vi "SVFA FFT Spectrum (Complex) (1 Ch).vi"(0 "scaled signal [EU]":waveform(dbl), 2 "window":T9=8 items=["None"=0, "Hanning"=1, "Hamming"=2, "Blackman-Harris"=3, "Exact Blackman"=4, "Blackman"=5, "Flat Top"=6, "4 Term B-Harris "=7, "7 Term B-Harris"=8, "Low Sidelobe"=9, "Force"=64, "Exponential"=65, "Blackman Nuttall"=11, "Triangle"=30, "Bartlett-Hanning"=31, "Bohman"=32, "Parzen"=33, "Welch"=34, "Kaiser"=60, "Dolph-Chebyshev"=61, "Gaussian"=62], 5 "error in":errorcluster, 7 "averaging parameters":T1={"averaging mode"=enum."No averaging", "weighting mode"=enum."Exponential", "number of averages"=10, "linear mode"=enum."One shot"} {"number of averages" min=1 step=1}, 9 "restart averaging (F)":bool) -> (11 "averaging done":bool, 13 "averages completed":dbl, 14 "complex spectrum":T8={"complex spectrum response"={"f0"=0.0, "df"=1.0, "complex spectrum"=[]}, "spectrum info"={"channel name"="", "description"="", "x-axis units"=0, "spectral info"={"spectrum type"=enum."Power [Magnitude^2]", "linear/dB"=enum."linear", "window"=0, "window size"=0, "FFT size"=0}, "engineering units"=0, "custom label"="", "dB reference [EU]"=0.0, "peak units"=enum."rms", "weighting filter"=0, "spectral density?"=FALSE, "unit label"="", "spectrum skewed?"=FALSE, "complimentary spectrum units"=enum."none"}} {"spectrum info"."x-axis units" items=["Time (s)"=0, "Frequency-CB (Hz)"=1, "Frequency-CPB (Hz)"=1248, "Frequency-Arbitrary (Hz)"=2357, "Quefrency (s)"=2, "Revolutions (rev)"=3, "Order"=4, "Speed (RPM)"=11, "Speed (rad/s)"=21, "Index"=65535]; "spectrum info"."weighting filter" items=["Linear", "A-weighting", "B-weighting", "C-weighting", "ITU-R 468-4", "Dolby", "CCITT", "C-message", "Wb", "Wc", "Wd", "We", "Wf", "Wh", "Wj", "Wk", "Wm", "AES17 20 kHz lowpass", "AES17 40 kHz lowpass", "AES17 20 kHz highpass", "AES17 40 kHz highpass"]; "spectrum info"."dB reference [EU]" format="%.2f"; "spectrum info"."engineering units" items=["custom..."=0, "V"=1, "A"=21, "C"=30, "pC"=31, "s"=32, "-"=29, "Pa"=2, "N"=20, "g"=3, "m/s^2"=4, "m/s"=5, "m"=6, "mm/s"=12, "mm"=13, "micron/s"=14, "micron"=15, "in/s^2"=7, "in/s"=8, "in"=9, "mil/s"=10, "mil"=11, "rad/s^2"=16, "rad/s"=17, "rad"=18, "deg/s^2"=26, "deg/s"=27, "deg"=28, "RPM"=22, "cycle/s^2"=23, "Hz"=24, "cycle"=25, "strain"=19]; "spectrum info"."spectral info"."window" items=["None "=0, "Hanning"=1, "Hamming"=2, "Blackman-Harris"=3, "Exact Blackman"=4, "Blackman"=5, "Flat Top"=6, "4 Term B-Harris "=7, "7 Term B-Harris"=8, "Low Sidelobe"=9, "Force - Exponential"=10, "Gaussian"=62]; "complex spectrum response"."complex spectrum" format="%.2f"; "complex spectrum response"."df" format="%.2f"; "complex spectrum response"."f0" format="%.2f"}, 19 "error out":errorcluster)   [LabVIEW 2017]
doc: "Computes the Fast Fourier Transform (FFT) spectrum of <B>scaled signal [EU]</B>. This VI returns FFT results as the complex form of the FFT spectrum. Wire data to the <B>scaled signal [EU]</B> input to determine the polymorphic instance to use or manually select the instance."
uses:
  <vilib>/addons/_NISVFA/_Shared subVIs/Controls/svc_Window.ctl
  <vilib>/addons/_NISVFA/_Shared subVIs/Controls/svc_Spectrum Info.ctl
  <vilib>/addons/_NISVFA/_Shared subVIs/Controls/svc_X-Axis Units.ctl
  <vilib>/addons/_NISVFA/_Shared subVIs/Controls/svc_Spectrum Type.ctl
  <vilib>/addons/_NISVFA/_Shared subVIs/Controls/svc_Engineering Units Text Ring.ctl
  <vilib>/addons/_NISVFA/_Shared subVIs/Controls/svc_Weighting Filter Text Ring.ctl
  <vilib>/addons/_NISVFA/_Shared subVIs/Controls/svc_Complimentary Spectrum Units.ctl
  <vilib>/Analysis/2dsp.llb/Real FFT.vi
  <vilib>/Analysis/2dsp.llb/Power Spectrum (DBL).vi
  <vilib>/addons/_NISVFA/_Shared subVIs/Spectrum Averaging/svfa_No Average Array (complex).vi
  <vilib>/addons/_NISVFA/_Shared subVIs/Spectrum Averaging/svfa_Average Array (complex).vi
  <vilib>/addons/_NISVFA/_Shared subVIs/Common/sv_Get NI Property Name String.vi
  <vilib>/addons/_NISVFA/_Shared subVIs/Spectrum Averaging/svfa_No Average Array (real).vi
  <vilib>/addons/_NISVFA/_Shared subVIs/Spectrum Averaging/svfa_Average Array (real).vi
  <vilib>/addons/_NISVFA/_Shared subVIs/Spectrum Averaging/svfa_Peak Hold Array.vi
  <vilib>/addons/_NISVFA/_Shared subVIs/Windowing/svfa_Scaled Time Domain Window (Array).vi
  <vilib>/addons/_NISVFA/_Shared subVIs/Common/svc_Get SV Channel Info.vi
  <vilib>/addons/_NISVFA/_Shared subVIs/Common/svc_Spectrum Units.vi
  <vilib>/Analysis/4window.llb/Force Window.vi
  <vilib>/Analysis/4window.llb/Force Window (DBL).vi
  <vilib>/Analysis/4window.llb/Exponential Window.vi
  <vilib>/Analysis/4window.llb/Exponential Window (DBL).vi
  <vilib>/addons/_NISVFA/_Shared subVIs/Spectrum Info/sfva_Set SV Info in Spectrum Info Description.vi
  <vilib>/addons/_NISVFA/_Shared subVIs/Spectrum Info/sfva_Get SV Info from Spectrum Info Description.vi
  <vilib>/addons/_NISVFA/_Shared subVIs/Common/svc_Get Weighting Enum and Labels.vi
  <vilib>/addons/_NISVFA/_Shared subVIs/Common/svc_Unit Label Lexical Class.vi
  <vilib>/addons/_NISVFA/_Shared subVIs/Common/svc_Engineering Units to Unit Label.vi
  <vilib>/addons/_NISVFA/_Shared subVIs/Common/svc_Format Value (DBL).vi
  <vilib>/addons/_NISVFA/_Shared subVIs/Common/svc_Channel Info to Spectrum Info.vi
  <vilib>/addons/_NISVFA/_Shared subVIs/Common/svc_Unit Label to Engineering Units.vi
  <vilib>/Utility/error.llb/Error Cluster From Error Code.vi
  <vilib>/Analysis/0measdsp.llb/Scaled Time Domain Window.vi
  <vilib>/Analysis/0measdsp.llb/Scaled Time Domain Window (DBL).vi
  <vilib>/addons/_NISVFA/_Spectrum Processing/subVIs/svfa_Spectrum Info Window to windowTd Type Def.vi
  <vilib>/addons/_NISVFA/_Shared subVIs/Common/svc_Window Parameters.vi
  <vilib>/addons/_NISVFA/_Shared subVIs/Common/svc_Get Window Info.vi
  <vilib>/Analysis/NI_AALPro.lvlib
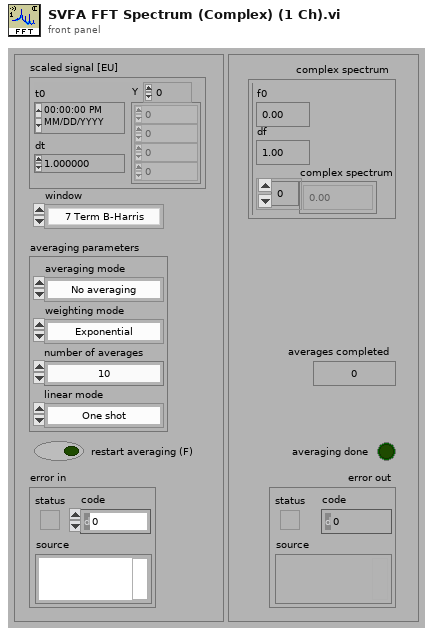
[diagram p1: front panel]
types:
  T1 = cluster{"averaging mode":enum16{"No averaging", "Vector averaging", "RMS averaging", "Peak hold"}, "weighting mode":enum16{"Linear", "Exponential"}, "number of averages":u32, "linear mode":enum16{"One shot", "Auto restart"}}
  T2 = typedef "svc_Spectrum Info.ctl" = cluster{"channel name":string, "description":string, "x-axis units":T3, "spectral info":cluster{"spectrum type":T4, "linear/dB":enum16{"linear", "dB"}, "window":u16, "window size":i32, "FFT size":i32}, "engineering units":T5, "custom label":string, "dB reference [EU]":dbl, "peak units":enum16{"rms", "peak", "peak-peak"}, "weighting filter":T6, "spectral density?":bool, "unit label":string, "spectrum skewed?":bool, "complimentary spectrum units":T7}
  T3 = typedef "svc_X-Axis Units.ctl" = u16
  T4 = typedef "svc_Spectrum Type.ctl" = enum16{"FFT Spectrum [complex]", "Amplitude [Magnitude]", "Power [Magnitude^2]", "Cross Spectrum [complex]", "Frequency Response [Complex]"}
  T5 = typedef "svc_Engineering Units Text Ring.ctl" = u16
  T6 = typedef "svc_Weighting Filter Text Ring.ctl" = u16
  T7 = typedef "svc_Complimentary Spectrum Units.ctl" = enum16{"none", "radians", "degrees", "cycles", "imaginary"}
  T8 = cluster{"complex spectrum response":cluster{"f0":dbl, "df":dbl, "complex spectrum":cdb[]}, "spectrum info":T2}
  T9 = typedef "svc_Window.ctl" = u32
  T10 = enum16{"Restart processing", "Continue processing", "Skip processing"}
  T11 = cluster{"complex FFT":cdb[], "Mag/Real FFT":dbl[], "f0":dbl, "df":dbl, "averages completed":dbl, "averaging parameters":cluster{"averaging mode":enum16{"No averaging", "Vector averaging", "RMS averaging", "Peak hold"}, "weighting mode":enum16{"Linear", "Exponential"}, "number of averages":u32, "linear mode":enum16{"One shot", "Auto restart"}}}
  T12 = enum16{"No averaging", "Vector averaging", "RMS averaging", "Peak hold"}
  T13 = cluster{"complex FFT":cdb[], "real FFT":dbl[], "f0":dbl, "df":dbl, "averages completed":dbl, "averaging parameters":cluster{"averaging mode":enum16{"No averaging", "Vector averaging", "RMS averaging", "Peak hold"}, "weighting mode":enum16{"Linear", "Exponential"}, "number of averages":u32, "linear mode":enum16{"One shot", "Auto restart"}}}
  T14 = cluster{"complex spectrum":cluster{"f0":dbl, "df":dbl, "complex spectrum":cdb[]}, "spectrum info":T2}
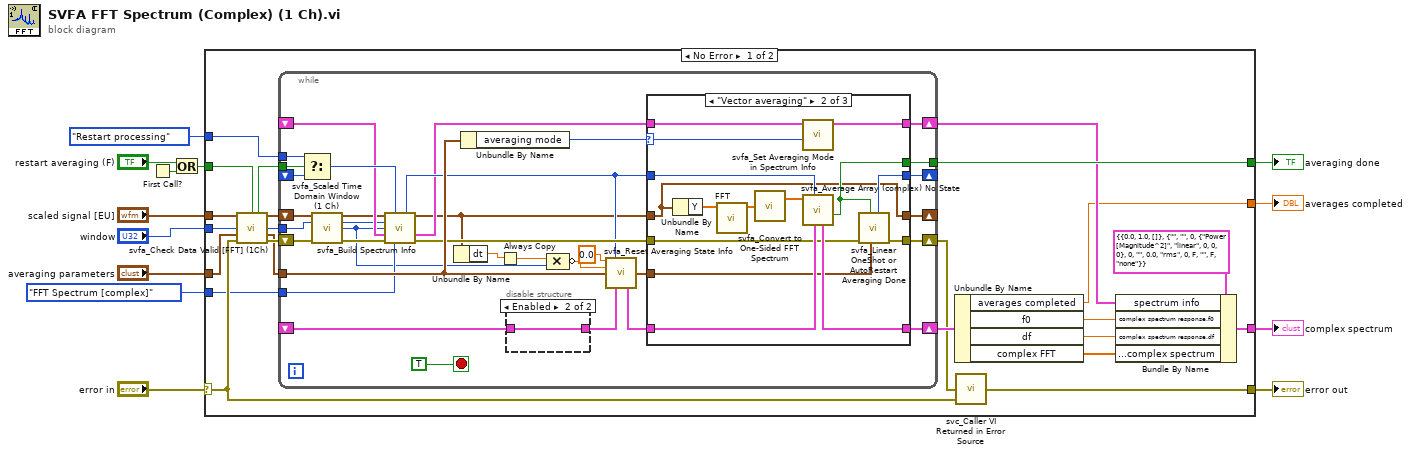
[diagram p0: block diagram]
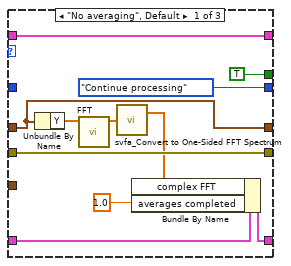
[diagram p2: hidden frame]
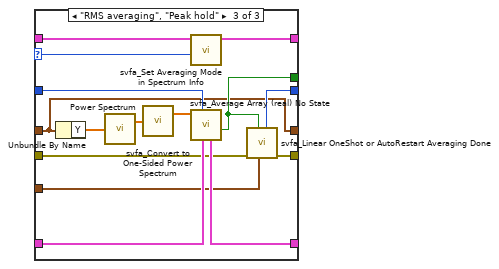
[diagram p3: hidden frame]
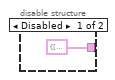
[diagram p4: hidden frame]
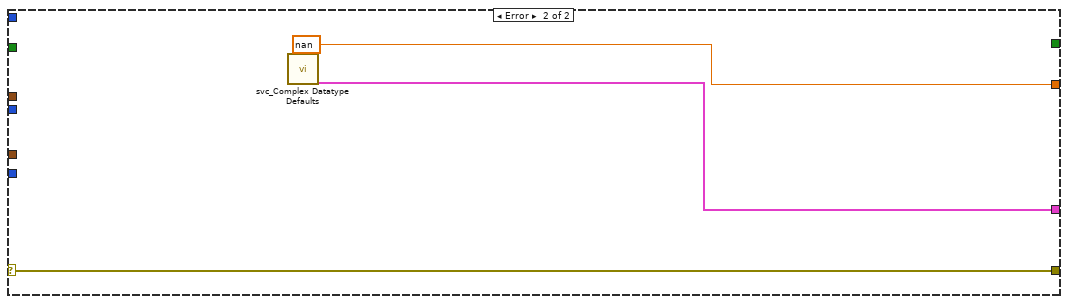
[diagram p5: hidden frame]
diagram:
  n1 = First Call?() -> (First Call?: T/F=w5:bool)
  n2 = Or(x="restart averaging (F)", y=w5) -> (x .or. y?=w3:bool)
  n3 = case shown="No Error" "error in" {
    selector: "error in" -> [w31 w115]
    tunnel: "window" -> [w35 _]
    tunnel: "averaging parameters" -> [w34 _]
    tunnel: [w32 w115] -> w13
    tunnel: "scaled signal [EU]" -> [w36 _]
    tunnel: w3 -> [w33 _]
    tunnel: [w16 nan ("averages completed")] -> w8
    tunnel: [w25 _] -> w7
    tunnel: [w23 w113] -> w6
    tunnel: T10."Restart processing" ("t") -> [w15 _]
    tunnel: svc_Spectrum_Type."FFT Spectrum [complex]" ("spectrum type") -> [w14 _]
    frame No Error {
      n4 = call <vilib>:"svfa_Check Data Valid [FFT] (1Ch).vi"("signal in [X]"=w36, "restart averaging (F)"=w33, "window"=w35, "averaging parameters"=w34, "error in (no error)"=w31) -> ("restart averaging"=w30:bool, "dup signal in [X]"=w29:waveform(dbl), "dup window"=w26:T9, "dup averaging parameters"=w27:T1, "error out"=w28:errorcluster)  [unwired: 6 in]
      n5 = while {
        shift-left: _ -> [w57]
        shift-right: [w66] -> w22
        tunnel: w30 -> [w65]
        tunnel: [w70] -> w25
        shift-right: [w47] -> _
        shift-left: _ -> [w64]
        shift-right: [w40] -> w21
        shift-left: _ -> [w62]
        tunnel: w15 -> [w61]
        tunnel: w27 -> [w60]
        tunnel: w26 -> [w59]
        shift-right: [w45] -> w17
        shift-left: w28 -> [w68]
        shift-right: [w38] -> _
        shift-left: w29 -> [w69]
        tunnel: w14 -> [w42]
        stop <- TRUE stop-if-true
        n6 = Select(t=w61, s=w65, f=w64) -> (s? t:f=w63:T10)
        n7 = call <vilib>:"svfa_Scaled Time Domain Window (1 Ch).vi"("Signal in [X]"=w69, "window"=w59, "error in"=w68) -> ("Windowed Waveform"=w53:waveform(dbl), "dup window"=w52:T9, "window length"=w39:i32, "error out"=w55:errorcluster)  [unwired: 7 in, 2 out]
        n8 = call <vilib>:"svfa_Build Spectrum Info.vi"("scaled signal [EU]"=w53, "processing control"=w63, "window"=w52, "window size"=w39, "spectrum info in"=w62, "error in (no error)"=w55, "spectrum type"=w42) -> ("dup processing control"=w50:T10, "dup scaled signal [EU]"=w37:waveform(dbl), "spectrum info out"=w41:T2, "error out"=w54:errorcluster)  [unwired: 5 in]
        n9 = Unbundle By Name ("Get Waveform Components")(w37) -> ("dt"=w48:dbl)
        n10 = Unbundle By Name(w60) -> ("averaging mode"=w56:T12)
        n11 = Always Copy(1:w48) -> (0:w43:dbl)
        n12 = disable-structure shown="Enabled" {
          disable-tunnel: [T11 {"complex FFT"=[], "Mag/Real FFT"=[], "f0"=0.0, "df"=0.0, "averages completed"=0.0, "averaging parameters"={"averaging mode"=enum."No averaging", "weighting mode"=enum."Linear", "number of averages"=0, "linear mode"=enum."One shot"}} ("averaging state info out") w112] -> w58
          disable-tunnel: w57 -> [_ w112]
          frame Disabled {
          }
          frame Enabled {
          }
        }
        n13 = Compound Arithmetic op=MULTIPLY(w43, w39) -> (invert w44:dbl)
        n14 = call <vilib>:"svfa_Reset Averaging State Info.vi"("f0"=0.0, "processing control"=w50, "df"=w44, "averaging parameters"=w60, "averaging state info in"=w58) -> ("dup averaging parameters"=w46:T1, "averaging state info out"=w49:T13)  [unwired: 9 in]
        n15 = case shown="\"Vector averaging\"" w56 {
          selector: w56 -> [_ w84 w99]
          tunnel: [w80 w91 w105] -> w45
          tunnel: [TRUE ("averaging done") w89 w104] -> w70
          tunnel: w54 -> [w80 w88 w105]
          tunnel: w50 -> [_ w96 w110]
          tunnel: [w78 w92 w106] -> w66
          tunnel: w49 -> [w79 w95 w109]
          tunnel: [T10."Continue processing" ("processing control") w90 w103] -> w47
          tunnel: w46 -> [_ w87 w102]
          tunnel: w41 -> [w73 w86 w101]
          tunnel: [w73 w85 w100] -> w40
          tunnel: w37 -> [w71 w82 w97]
          tunnel: [w71 w82 w97] -> w38
          frame "No averaging", Default {
            n16 = Unbundle By Name ("Get Waveform Components")(w71) -> ("Y"=w72:dbl[])
            n17 = call-poly <vilib>:"FFT.vi"("X"=w72) -> ("FFT {X}"=w77:cdb[])  [unwired: 9 in, 1 out]
            n18 = call <vilib>:"svfa_Convert to One-Sided FFT Spectrum.vi"("two-sided FFT spectrum"=w77) -> ("one-sided FFT spectrum"=w76:cdb[])  [unwired: 1 out]
            n19 = Bundle By Name(cluster=w79, "complex FFT"=w76, "averages completed"=1.0) -> (w78:T13)
          }
          frame "Vector averaging" {
            n20 = Unbundle By Name ("Get Waveform Components")(w82) -> ("Y"=w83:dbl[])
            n21 = call-poly <vilib>:"FFT.vi"("X"=w83) -> ("FFT {X}"=w94:cdb[])  [unwired: 9 in, 1 out]
            n22 = call <vilib>:"svfa_Convert to One-Sided FFT Spectrum.vi"("two-sided FFT spectrum"=w94) -> ("one-sided FFT spectrum"=w93:cdb[])  [unwired: 1 out]
            n23 = call <vilib>:"svfa_Set Averaging Mode in Spectrum Info.vi"("averaging mode"=w84, "spectrum info in"=w86) -> ("spectrum info out"=w85:T2)  [unwired: 8 in, 1 out]
            n24 = call <vilib>:"svfa_Average Array (complex) No State.vi"("averaging state info in"=w95, "processing control"=w96, "array"=w93) -> ("averaging done"=w89:bool, "averaging state info out"=w92:T11)  [unwired: 5 in, 2 out]
            n25 = call <vilib>:"svfa_Linear OneShot or AutoRestart Averaging Done.vi"("averaging parameters"=w87, "averaging done"=w89, "error in (no error)"=w88) -> ("error out"=w91:errorcluster, "processing control"=w90:T10)  [unwired: 7 in]
          }
          frame "RMS averaging", "Peak hold" {
            n26 = Unbundle By Name ("Get Waveform Components")(w97) -> ("Y"=w98:dbl[])
            n27 = call-poly <vilib>:"Power Spectrum.vi"("X"=w98) -> ("Power Spectrum"=w108:dbl[])  [unwired: 1 out]
            n28 = call <vilib>:"svfa_Convert to One-Sided Power Spectrum.vi"("two-sided power spectrum"=w108) -> ("one-sided power spectrum"=w107:dbl[])  [unwired: 1 out]
            n29 = call <vilib>:"svfa_Set Averaging Mode in Spectrum Info.vi"("averaging mode"=w99, "spectrum info in"=w101) -> ("spectrum info out"=w100:T2)  [unwired: 8 in, 1 out]
            n30 = call <vilib>:"svfa_Average Array (real) No State.vi"("averaging state info in"=w109, "processing control"=w110, "array"=w107) -> ("averaging done"=w104:bool, "averaging state info out"=w106:T11)  [unwired: 5 in, 2 out]
            n31 = call <vilib>:"svfa_Linear OneShot or AutoRestart Averaging Done.vi"("averaging parameters"=w102, "averaging done"=w104) -> ("processing control"=w103:T10)  [unwired: 8 in, 1 out]
          }
        }
      }
      n32 = Unbundle By Name(w22) -> ("averages completed"=w16:dbl, "f0"=w20:dbl, "df"=w19:dbl, "complex FFT"=w18:cdb[])
      n33 = call <vilib>:"svc_Caller VI Returned in Error Source.vi"("warning input to caller"=w31, "error in (no error)"=w17) -> ("error out"=w32:errorcluster)  [unwired: 3 in]
      n34 = Bundle By Name(cluster=T8 {"complex spectrum response"={"f0"=0.0, "df"=1.0, "complex spectrum"=[]}, "spectrum info"={"channel name"="", "description"="", "x-axis units"=0, "spectral info"={"spectrum type"=enum."Power [Magnitude^2]", "linear/dB"=enum."linear", "window"=0, "window size"=0, "FFT size"=0}, "engineering units"=0, "custom label"="", "dB reference [EU]"=0.0, "peak units"=enum."rms", "weighting filter"=0, "spectral density?"=FALSE, "unit label"="", "spectrum skewed?"=FALSE, "complimentary spectrum units"=enum."none"}} ("complex spectrum"), "spectrum info"=w21, "complex spectrum response.f0"=w20, "complex spectrum response.df"=w19, "complex spectrum response.complex spectrum"=w18) -> (w23:T8)
    }
    frame Error {
      n35 = call <vilib>:"svc_Complex Datatype Defaults.vi"() -> ("complex spectrum"=w113:T14)  [unwired: 11 in, 8 out]
    }
  }
  "error out" <- w13
  "complex spectrum" <- w6
  "averages completed" <- w8
  "averaging done" <- w7
